vi "HexToString.vi"(10 "字符个数":i32=6, 11 "数组":u16[](array[numeric]) format="%04xH") -> (3 "STRING":string[](array[string]))   [LabVIEW 2016, in "斯坦道多参数.lvlib"]
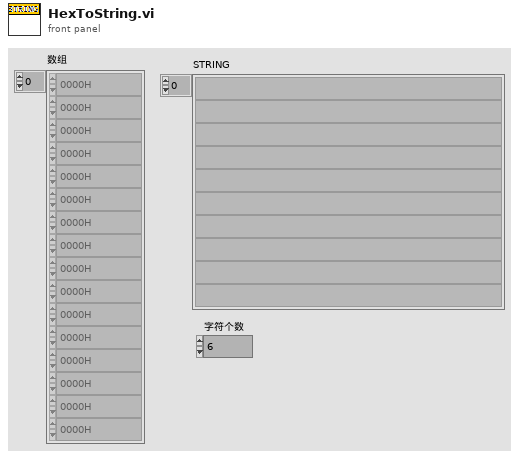
[diagram p1: front panel]
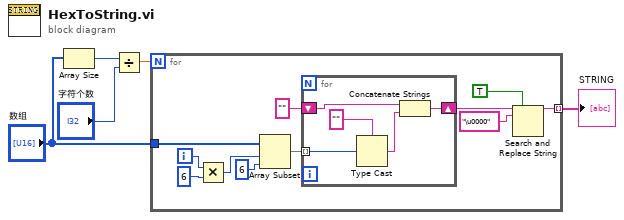
[diagram p0: block diagram]
diagram:
  n1 = Array Size(array="数组") -> (size(s)=w5:i32)
  n2 = Divide(x=w5, y="字符个数") -> (x/y=w3:dbl)
  n3 = for {
    N: w3 -> [_]
    tunnel: "数组" -> [w16]
    tunnel: [w8] -> w2 mode=indexing
    i -> [w15]
    n4 = Multiply(x=w15, y=6) -> (x*y=w12:i32)
    n5 = Array Subset(array=w16, index=w12, length=6 ("索引")) -> (w10:u16[])
    n6 = for {
      shift-right: [w21] -> w9
      shift-left: "" -> [w18]
      tunnel: w10 -> [w20] mode=indexing
      n7 = Type Cast(type="", x=w20) -> (*(type *) &x=w17:string)
      n8 = Concatenate Strings(w18, w17) -> (w21:string)
    }
    n9 = Search and Replace String(replace all?=TRUE ("替换全部？(F)"), input string=w9, search string="\u0000" ("搜索字符串")) -> (result string=w8:string)  [unwired: 5 in, 3 out]
  }
  "STRING" <- w2
